vi "Com Port Configuration.vi"(8 "error in":errorcluster, 11 "Com Port In":refnum<visa-resource-name>) -> (0 "error out":errorcluster, 3 "Com Port Out":refnum<visa-resource-name>)   [LabVIEW 2018]
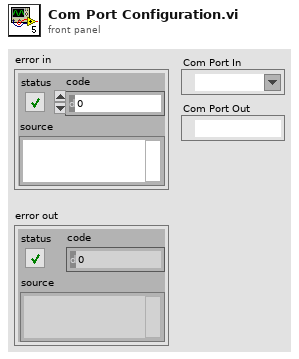
[diagram p1: front panel]
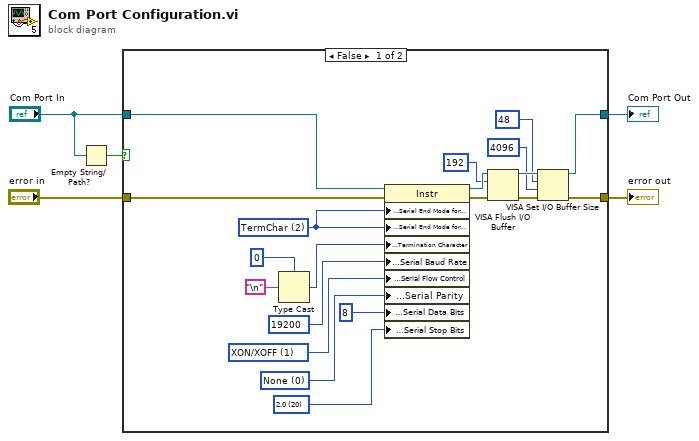
[diagram p0: block diagram]
diagram:
  n1 = Empty String/Path?(string/path="Com Port In") -> (empty?=w1:bool)
  n2 = case shown="False" w1 {
    tunnel: "Com Port In" -> [w9 w26]
    tunnel: "error in" -> [w8 w27]
    tunnel: [w7 w27] -> w4
    tunnel: [w6 w26] -> w3
    frame False {
      w11 = u16 20 items=["1.0"=10, "1.5"=15, "2.0"=20] ("Serial Settings:Stop Bits")
      w14 = u16 0 items=["None", "Odd", "Even", "Mark", "Space"] ("Serial Settings:Parity")
      w15 = u16 1 items=["None", "XON/XOFF", "RTS/CTS", "XON/XOFF & RTS/CTS", "DTR/DSR", "XON/XOFF & DTR/DSR"] ("Serial Settings:Flow Control")
      w16 = u16 2 items=["None", "LastBit", "TermChar"] ("Serial Settings:Serial End Mode for Reads")
      n3 = Type Cast(type=u8 0, x="\n" ("Line Feed Constant")) -> (*(type *) &x=w10:u8)
      n4 = property class="Instr"(reference=w9, error in=w8, "Serial Settings:Serial End Mode for Reads"=w16, "Serial Settings:Serial End Mode for Writes"=w16, "Message Based Settings:Termination Character"=w10, "Serial Settings:Serial Baud Rate"=u32 19200 ("Serial Settings:Baud Rate"), "Serial Settings:Serial Flow Control"=w15, "Serial Settings:Serial Parity"=w14, "Serial Settings:Serial Data Bits"=u16 8 ("Serial Settings:Data Bits"), "Serial Settings:Serial Stop Bits"=w11) -> (reference out=w22:refnum<visa-resource-name>, error out=w24:errorcluster)
      n5 = VISA Flush I/O Buffer(VISA resource name=w22, mask (16)=u16 192, error in (no error)=w24) -> (VISA resource name out=w25:refnum<visa-resource-name>, error out=w23:errorcluster)
      n6 = VISA Set I/O Buffer Size(VISA resource name=w25, mask (16)=u16 48, size (4096)=u32 4096 ("size (0)"), error in (no error)=w23) -> (VISA resource name out=w6:refnum<visa-resource-name>, error out=w7:errorcluster)
    }
    frame True {
    }
  }
  "error out" <- w4
  "Com Port Out" <- w3
